vi "solar_target2.vi"(11 "Target":string) -> ()   [LabVIEW 2018]
doc: "SOLAR target demo."
uses:
  solar/solar.lvclass
  solar/solar Msg EnQ (This).vi
  solar/solar Msg UE Generate.vi
  voyager/solar_voy_def/solar_voy_def Import (Variants).vi
  solar/solar Msg Voyager (TLM).vi
  qtimer/solar_qtimer_ctl QTimer Settings.ctl
panel:
  in  "Log_Write":string="Test"
  in  "Log Write":bool
  in  "Log Pause":bool
  in  "Log Restart":bool
  in  "QTimer Start Target":bool
  in  "QTimer Stop Target":bool
  in  "QTimer Target":string
  out "QTimers":T1[](array[typedef])
  out "Subscribed DATA":variant
  out "Subscribed MSG":string
  out "Packets out":T2={"MYUINT8"={"VALUE"=255}, "MYUINT16"={"VALUE"=65535}, "MYUINT32"={"VALUE"=4294967295}, "MYUINT64"={"VALUE"=18446744073709551615}, "MYINT8"={"VALUE"=-128}, "MYINT16"={"VALUE"=-32768}, "MYINT32"={"VALUE"=-2147483648}, "MYINT64"={"VALUE"=-9223372036854775808}, "MYFLOAT32"={"VALUE"=3.141563}, "MYFLOAT64"={"VALUE"=-1.234567891e-05}, "MYSTRING"={"VALUE"="Hello World"}, "MYBLOCK"={"VALUE,t=block"="Þ­¾ï"}, "MYUINT8_ENUM"={"VALUE"=enum."ITEM2"}, "MYUINT16_ENUM"={"VALUE"=enum."BIRD"}, "MYUINT32_ENUM"={"VALUE"=enum."joe"}, "MYBOOLEAN"={"VALUE,s=OFF|ON"=FALSE}, "MYPATH"={"VALUE"=path "C:/Data/test.txt"}, "MYSTRING_FIXED"={"VALUE,b=24"="CAR"}, "MYBLOCK_FIXED"={"VALUE,t=block,b=32"="\u0001\u0002\u0003\u0004"}} {"MYFLOAT64"."VALUE" format="%#.12g"; "MYFLOAT32"."VALUE" format="%#.6g"}
  in  "Packets in":T2={"MYUINT8"={"VALUE"=255}, "MYUINT16"={"VALUE"=65535}, "MYUINT32"={"VALUE"=4294967295}, "MYUINT64"={"VALUE"=18446744073709551615}, "MYINT8"={"VALUE"=-128}, "MYINT16"={"VALUE"=-32768}, "MYINT32"={"VALUE"=-2147483648}, "MYINT64"={"VALUE"=-9223372036854775808}, "MYFLOAT32"={"VALUE"=3.141563}, "MYFLOAT64"={"VALUE"=-1.234567891e-05}, "MYSTRING"={"VALUE"="Hello World"}, "MYBLOCK"={"VALUE,t=block"="Þ­¾ï"}, "MYUINT8_ENUM"={"VALUE"=enum."ITEM2"}, "MYUINT16_ENUM"={"VALUE"=enum."BIRD"}, "MYUINT32_ENUM"={"VALUE"=enum."joe"}, "MYBOOLEAN"={"VALUE,s=OFF|ON"=FALSE}, "MYPATH"={"VALUE"=path "C:/Data/test.txt"}, "MYSTRING_FIXED"={"VALUE,b=24"="CAR"}, "MYBLOCK_FIXED"={"VALUE,t=block,b=32"="\u0001\u0002\u0003\u0004"}} {"MYFLOAT64"."VALUE" format="%#.12g"; "MYFLOAT32"."VALUE" format="%#.6g"}
  out "Time":timestamp
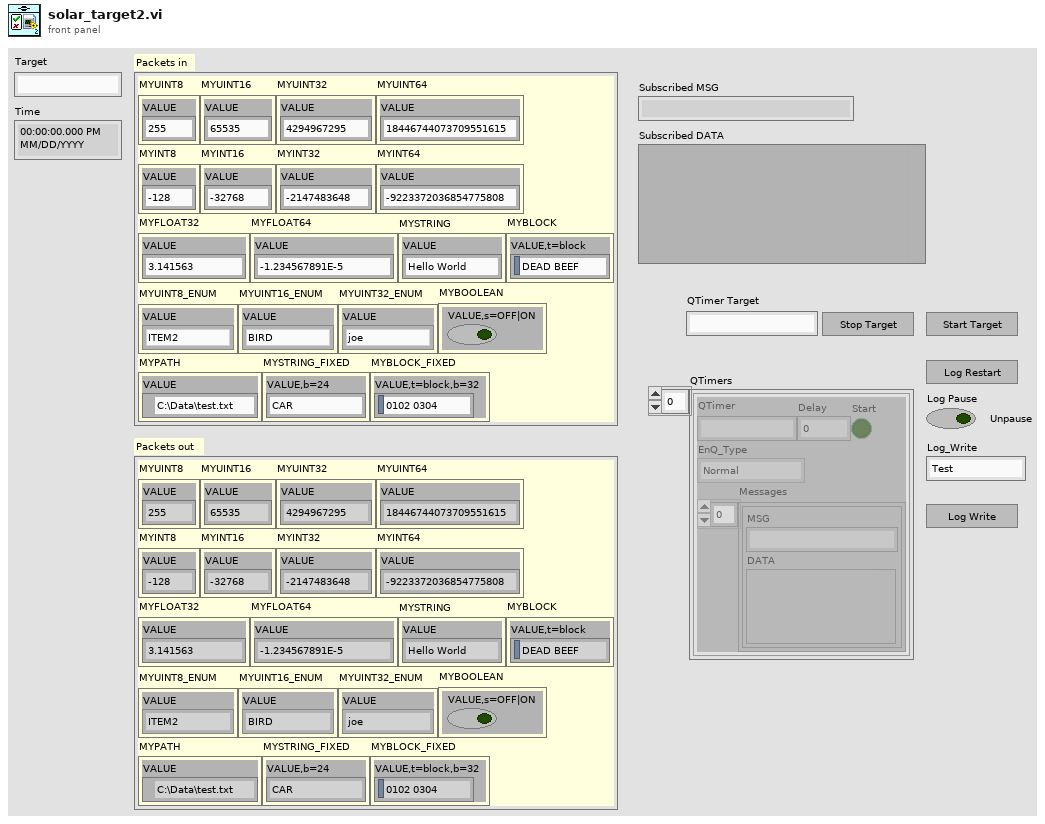
[diagram p1: front panel]
types:
  T1 = typedef "solar_qtimer_ctl QTimer Settings.ctl" = cluster{"QTimer":string, "Delay":i32, "Start":bool, "EnQ_Type":enum8{"Normal", "Priority", "IgnoreIfExists"}, "Messages":cluster{"MSG":string, "DATA":variant}[]}
  T2 = cluster{"MYUINT8":cluster{"VALUE":u8}, "MYUINT16":cluster{"VALUE":u16}, "MYUINT32":cluster{"VALUE":u32}, "MYUINT64":cluster{"VALUE":u64}, "MYINT8":cluster{"VALUE":i8}, "MYINT16":cluster{"VALUE":i16}, "MYINT32":cluster{"VALUE":i32}, "MYINT64":cluster{"VALUE":i64}, "MYFLOAT32":cluster{"VALUE":sgl}, "MYFLOAT64":cluster{"VALUE":dbl}, "MYSTRING":cluster{"VALUE":string}, "MYBLOCK":cluster{"VALUE,t=block":string}, "MYUINT8_ENUM":cluster{"VALUE":enum8{"ITEM1", "ITEM2", "ITEM3"}}, "MYUINT16_ENUM":cluster{"VALUE":enum16{"CAT", "DOG", "BIRD", "MOOSE"}}, "MYUINT32_ENUM":cluster{"VALUE":enum32{"ryan", "susan", "steve", "larry", "smith", "joe"}}, "MYBOOLEAN":cluster{"VALUE,s=OFF|ON":bool}, "MYPATH":cluster{"VALUE":path}, "MYSTRING_FIXED":cluster{"VALUE,b=24":string}, "MYBLOCK_FIXED":cluster{"VALUE,t=block,b=32":string}}
  T3 = cluster{"SIGNAL,s=NO|YES":bool, "VI,b=2048":string, "CONTROL,b=2048":string, "VALUE,t=block":string}
  T4 = cluster{"VALUE":enum8{"ITEM1", "ITEM2", "ITEM3"}}
  T5 = cluster{"VALUE":enum16{"CAT", "DOG", "BIRD", "MOOSE"}}
  T6 = cluster{"VALUE":enum32{"ryan", "susan", "steve", "larry", "smith", "joe"}}
  T7 = typedef "solar_voy_def_ctl PACKET.ctl" = cluster{"PACKET_ID":T8, "ENDIAN":enum8{"BIG", "LITTLE"}, "DESC":string, "HZRD":bool, "ITEMS":T9[], "NoExport":bool, "last_time":timestamp, "last_count":u32, "last_data":string}
  T8 = typedef "solar_voy_def_ctl PACKET_ID.ctl" = cluster{"ID":u16, "CMD":enum8{"CMD", "TLM"}, "TARGET":string, "PACKET":string}
  T9 = typedef "solar_voy_def_ctl ITEM.ctl" = cluster{"NAME":string, "OFFSET":i32, "SIZE":i32, "TYPE":T10, "EACH_SIZE":i32, "LVTYPE":T11, "MIN":dbl, "MAX":dbl, "DEFAULT":string, "DESC":string, "ID":bool, "MODIFIERS":variant, "last_value":variant}
  T10 = typedef "solar_voy_def_ctl ITEM TYPE.ctl" = enum8{"BLOCK", "INT", "UINT", "FLOAT", "STRING"}
  T11 = typedef "solar_type Item Type.ctl" = enum16{"NULL", "UNKNOWN", "CLUSTER", "I8", "I16", "I32", "I64", "U8", "U16", "U32", "U64", "U8_ENUM", "U16_ENUM", "U32_ENUM", "SGL", "DBL", "BOOLEAN", "STRING", "PATH", "VISA", "TAG", "TIME", "I8_1D", "I16_1D", "I32_1D", "I64_1D", "U8_1D", "U16_1D", "U32_1D", "U64_1D", "U8_ENUM_1D", "U16_ENUM_1D", "U32_ENUM_1D", "SGL_1D", "DBL_1D", "BOOLEAN_1D", "STRING_1D", "PATH_1D", "VISA_1D", "TAG_1D", "TIME_1D", "I8_2D", "I16_2D", "I32_2D", "I64_2D", "U8_2D", "U16_2D", "U32_2D", "U64_2D", "U8_ENUM_2D", "U16_ENUM_2D", "U32_ENUM_2D", "SGL_2D", "DBL_2D", "BOOLEAN_2D", "STRING_2D", "PATH_2D", "VISA_2D", "TAG_2D", "TIME_2D"}
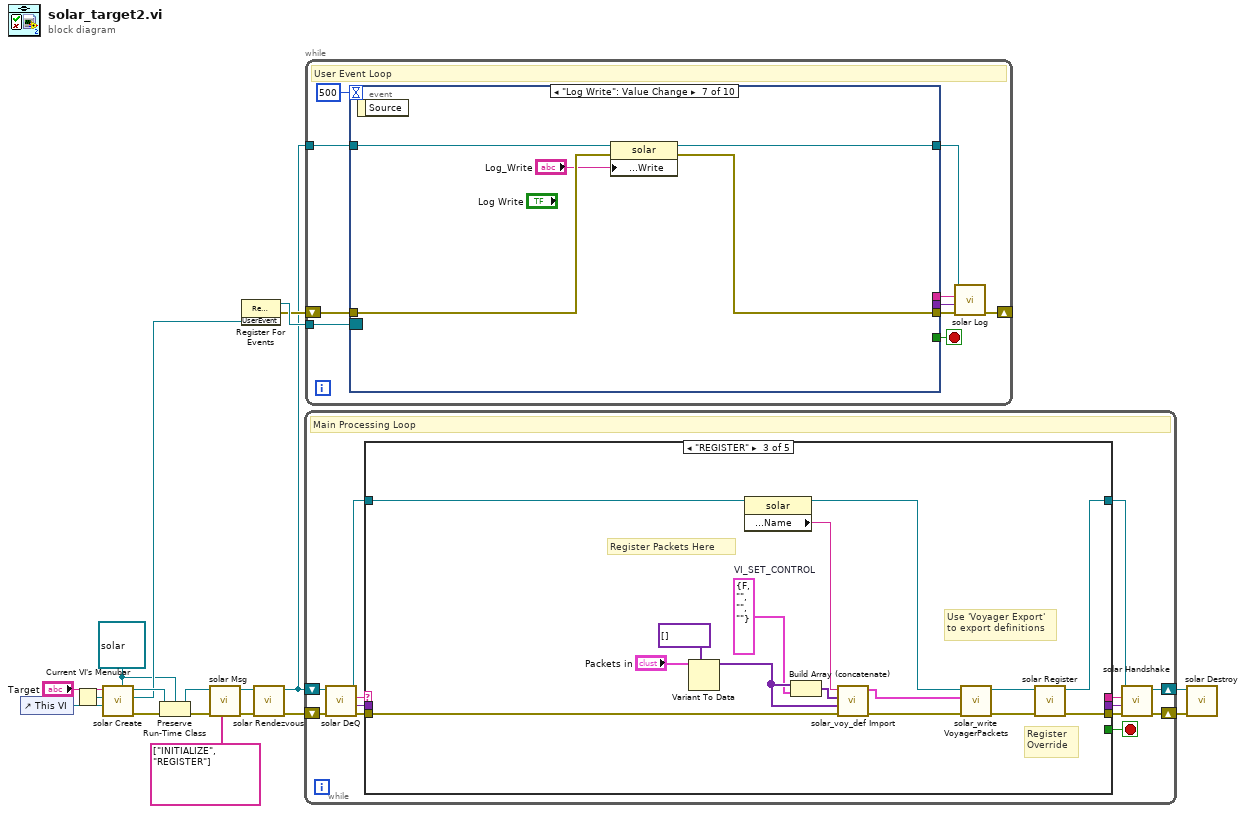
[diagram p0: block diagram]
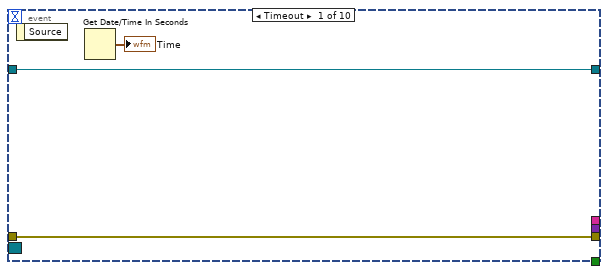
[diagram p2: hidden frame]
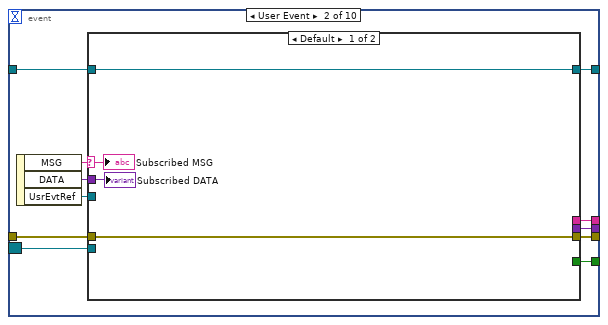
[diagram p3: hidden frame]
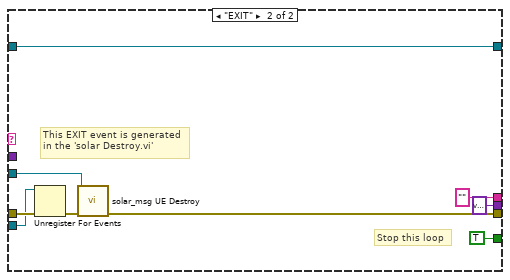
[diagram p4: hidden frame]
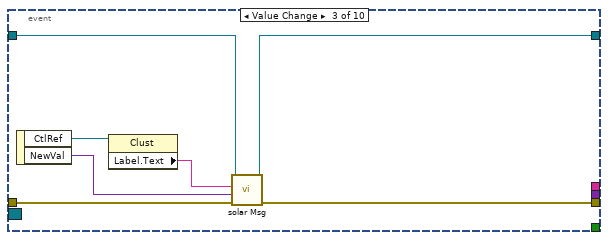
[diagram p5: hidden frame]
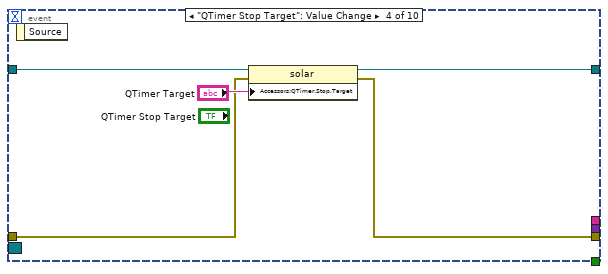
[diagram p6: hidden frame]
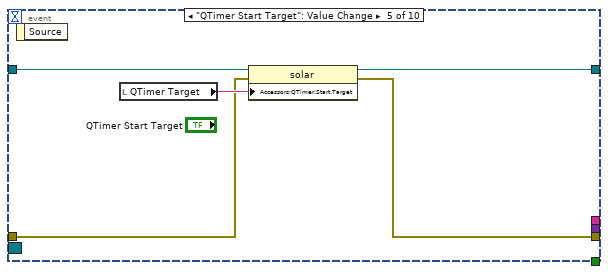
[diagram p7: hidden frame]
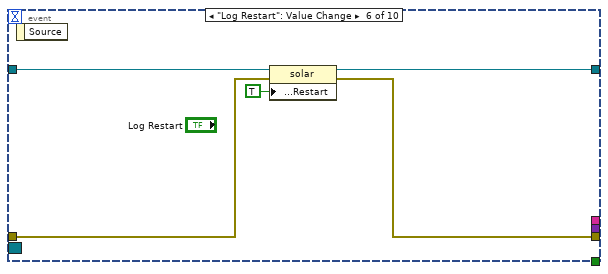
[diagram p8: hidden frame]
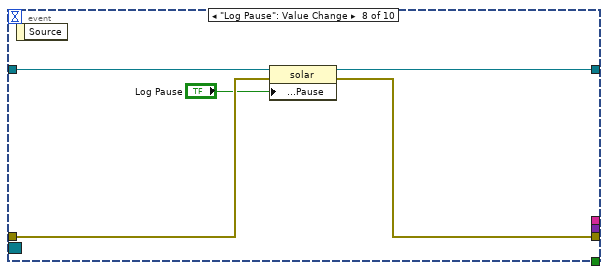
[diagram p9: hidden frame]
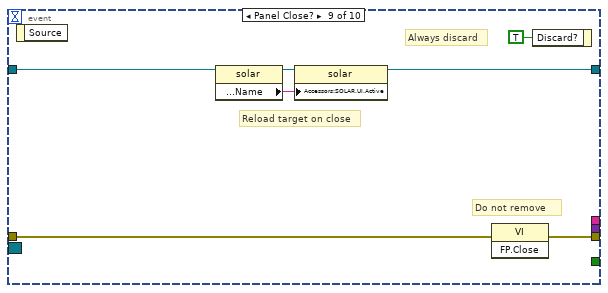
[diagram p10: hidden frame]
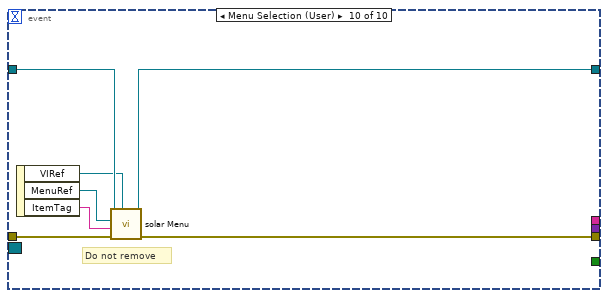
[diagram p11: hidden frame]
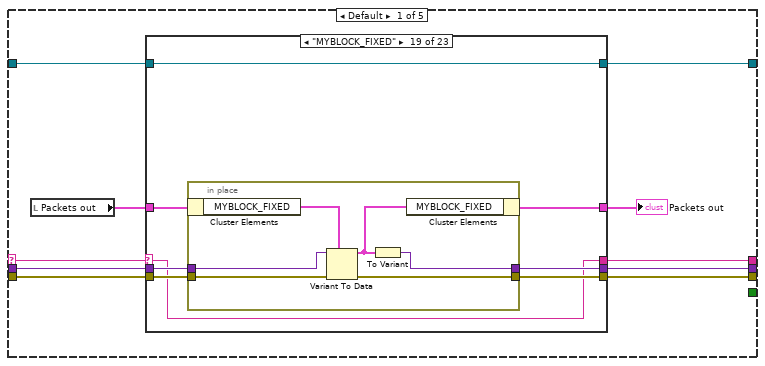
[diagram p12: hidden frame]
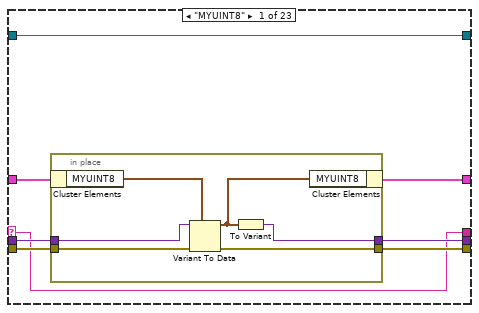
[diagram p13: hidden frame]
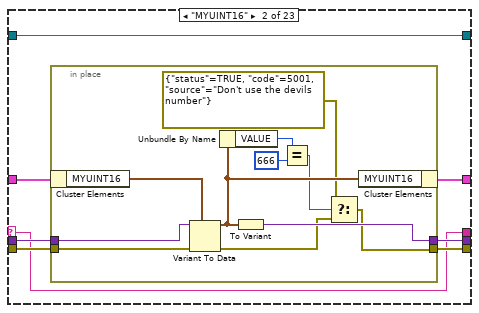
[diagram p14: hidden frame]
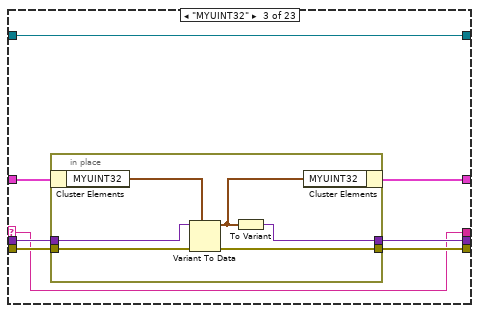
[diagram p15: hidden frame]
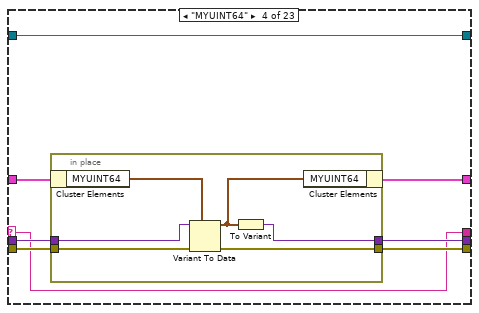
[diagram p16: hidden frame]
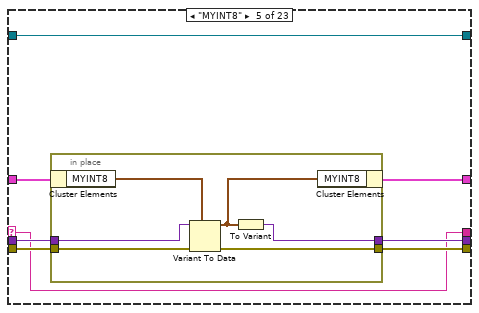
[diagram p17: hidden frame]
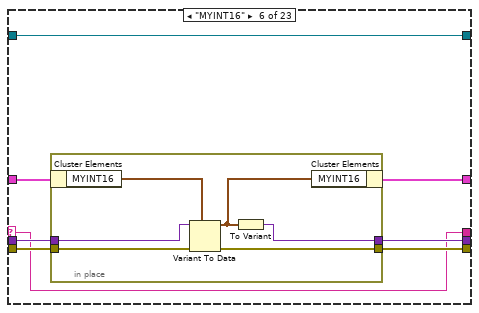
[diagram p18: hidden frame]
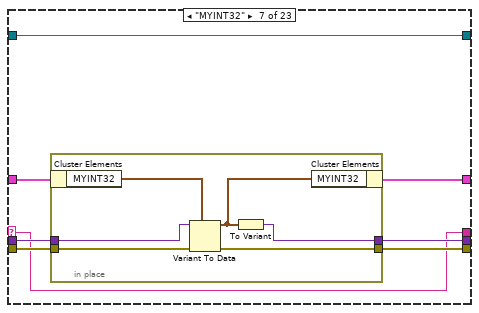
[diagram p19: hidden frame]
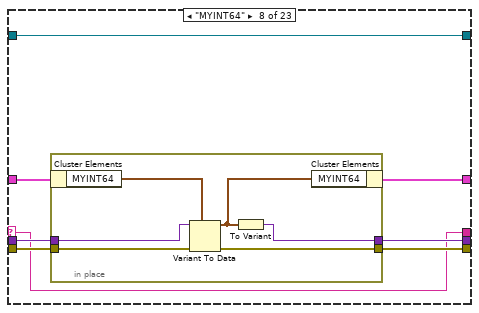
[diagram p20: hidden frame]
diagram:
  w11 = refnum<class "solar.lvclass"> refnum ("Default LVClass")
  n1 = control-ref of="This VI"() -> (w13:refnum<vi>)
  n2 = Current VI's Menubar() -> (w9:refnum<k9>)
  n3 = call "solar Create.vi"("Default LVClass"=w11, "VI Refnum"=w13, "VI MenuRef"=w9, "Target"="Target") -> ("error out"=w7:errorcluster, "UserEvent"=w14:refnum<user-event>, "solar"=w18:refnum<class "solar.lvclass">)  [unwired: 4 in, 1 out]
  n4 = Preserve Run-Time Class(object in=w18, error in=w7, 2:w11) -> (object out=w2:refnum<class "solar.lvclass">, error out=w3:errorcluster)
  n5 = call-poly "solar Msg.vi"("MSG Array"=string[] ["INITIALIZE", "REGISTER"] ("Script (\"PACKET{ITEM:VAL}\")"), "error in (no error)"=w3, "solar in"=w2) -> ("error out"=w6:errorcluster, "solar out"=w4:refnum<class "solar.lvclass">)  [unwired: 6 in, 1 out]
  n6 = register-events(w14) -> (reference out=w15:refnum<event-registration>, error out=w8:errorcluster)  [unwired: 2 in]
  n7 = call-dynamic "solar Rendezvous.vi"("error in (no error)"=w6, "solar in"=w4) -> ("error out"=w5:errorcluster, "solar out"=w1:refnum<class "solar.lvclass">)  [unwired: 6 in, 2 out]
  n8 = while {
    shift-right: [w28] -> w17
    shift-left: w5 -> [w30]
    shift-right: [w24] -> w16
    shift-left: w1 -> [w31]
    stop <- w23 stop-if-true
    # "Main Processing Loop"
    n9 = call "solar DeQ.vi"("error in (no error)"=w30, "solar in"=w31) -> ("error out"=w29:errorcluster, "DATA"=w19:variant, "MSG"=w20:string, "solar out"=w25:refnum<class "solar.lvclass">)  [unwired: 5 in, 1 out]
    n10 = case shown="\"REGISTER\"" w20 {
      selector: w20 -> [w36 _ _ _ _]
      tunnel: [w41 w367 w380 w386 w404] -> w27
      tunnel: w29 -> [w34 w360 w382 w390 w404]
      tunnel: [w39 w366 w379 w385 w405] -> w26
      tunnel: w25 -> [w40 w363 w373 w389 w405]
      tunnel: w19 -> [w35 _ _ _ _]
      tunnel: [_ _ _ w383 _] -> w23
      tunnel: [w38 _ _ _ _] -> w22
      tunnel: [w37 _ _ _ _] -> w21
      frame Default {
        n11 = local read "Packets out"() -> (w32:T2)
        n12 = case shown="\"MYBLOCK_FIXED\"" w36 {
          selector: w36 -> [w44 w58 w77 w91 w105 w119 w133 w147 w161 w175 w189 w203 w217 w231 w245 w259 w273 w287 w301 _ _ _ w338]
          tunnel: [w46 w60 w79 w93 w107 w121 w135 w149 w163 w177 w191 w205 w219 w233 w247 w261 w275 w289 w303 w315 w323 w330 w343] -> w41
          tunnel: w40 -> [w49 w63 w82 w96 w110 w124 w138 w152 w166 w180 w194 w208 w222 w236 w250 w264 w278 w292 w306 w319 w322 w329 w342]
          tunnel: [w49 w63 w82 w96 w110 w124 w138 w152 w166 w180 w194 w208 w222 w236 w250 w264 w278 w292 w306 w319 w321 w328 w341] -> w39
          tunnel: [w44 w58 w77 w91 w105 w119 w133 w147 w161 w175 w189 w203 w217 w231 w245 w259 w273 w287 w301 _ _ _ w340] -> w38
          tunnel: [w45 w59 w78 w92 w106 w120 w134 w148 w162 w176 w190 w204 w218 w232 w246 w260 w274 w288 w302 _ _ _ w339] -> w37
          tunnel: w35 -> [w47 w61 w80 w94 w108 w122 w136 w150 w164 w178 w192 w206 w220 w234 w248 w262 w276 w290 w304 w316 _ _ w337]
          tunnel: w34 -> [w48 w62 w81 w95 w109 w123 w137 w151 w165 w179 w193 w207 w221 w235 w249 w263 w277 w291 w305 w318 w324 w331 w336]
          tunnel: [w42 w56 w75 w89 w103 w117 w131 w145 w159 w173 w187 w201 w215 w229 w243 w257 w271 w285 w299 w320 w327 w334 w335] -> w33
          tunnel: w32 -> [w43 w57 w76 w90 w104 w118 w132 w146 w160 w174 w188 w202 w216 w230 w244 w258 w272 w286 w300 w320 w327 w334 w335]
          frame "MYUINT8" {
            n13 = in-place {
              in-place-border: w48 -> [w55]
              in-place-border: w47 -> [w54]
              in-place-border: [w51] -> w46
              in-place-border: [w50] -> w45
              n14 = in-place-cluster #1(w43) -> ("MYUINT8"=w53:cluster{"VALUE":u8})
              n15 = Variant To Data(error in=w55, type=w53, Variant=w54) -> (data=w52:cluster{"VALUE":u8}, error out=w51:errorcluster)
              n16 = To Variant(anything=w52) -> (Variant=w50:variant)
              n17 = in-place-cluster #1("MYUINT8"=w52) -> (w42:T2)
            }
          }
          frame "MYUINT16" {
            n18 = in-place {
              in-place-border: w62 -> [w74]
              in-place-border: w61 -> [w73]
              in-place-border: [w65] -> w60
              in-place-border: [w71] -> w59
              n19 = in-place-cluster #2(w57) -> ("MYUINT16"=w72:cluster{"VALUE":u16})
              n20 = Variant To Data(error in=w74, type=w72, Variant=w73) -> (data=w70:cluster{"VALUE":u16}, error out=w66:errorcluster)
              n21 = Unbundle By Name(w70) -> ("VALUE"=w69:u16)
              n22 = To Variant(anything=w70) -> (Variant=w71:variant)
              n23 = Equal?(x=w69, y=u16 666 ("VALUE")) -> (x = y?=w67:bool)
              n24 = Select(t=errorcluster {"status"=TRUE, "code"=5001, "source"="Don't use the devils number"}, s=w67, f=w66) -> (s? t:f=w65:errorcluster)
              n25 = in-place-cluster #2("MYUINT16"=w70) -> (w56:T2)
            }
          }
          frame "MYUINT32" {
            n26 = in-place {
              in-place-border: w81 -> [w88]
              in-place-border: w80 -> [w87]
              in-place-border: [w84] -> w79
              in-place-border: [w83] -> w78
              n27 = in-place-cluster #3(w76) -> ("MYUINT32"=w86:cluster{"VALUE":u32})
              n28 = Variant To Data(error in=w88, type=w86, Variant=w87) -> (data=w85:cluster{"VALUE":u32}, error out=w84:errorcluster)
              n29 = To Variant(anything=w85) -> (Variant=w83:variant)
              n30 = in-place-cluster #3("MYUINT32"=w85) -> (w75:T2)
            }
          }
          frame "MYUINT64" {
            n31 = in-place {
              in-place-border: w95 -> [w102]
              in-place-border: w94 -> [w101]
              in-place-border: [w98] -> w93
              in-place-border: [w97] -> w92
              n32 = in-place-cluster #4(w90) -> ("MYUINT64"=w100:cluster{"VALUE":u64})
              n33 = Variant To Data(error in=w102, type=w100, Variant=w101) -> (data=w99:cluster{"VALUE":u64}, error out=w98:errorcluster)
              n34 = To Variant(anything=w99) -> (Variant=w97:variant)
              n35 = in-place-cluster #4("MYUINT64"=w99) -> (w89:T2)
            }
          }
          frame "MYINT8" {
            n36 = in-place {
              in-place-border: w109 -> [w116]
              in-place-border: w108 -> [w115]
              in-place-border: [w112] -> w107
              in-place-border: [w111] -> w106
              n37 = in-place-cluster #5(w104) -> ("MYINT8"=w114:cluster{"VALUE":i8})
              n38 = Variant To Data(error in=w116, type=w114, Variant=w115) -> (data=w113:cluster{"VALUE":i8}, error out=w112:errorcluster)
              n39 = To Variant(anything=w113) -> (Variant=w111:variant)
              n40 = in-place-cluster #5("MYINT8"=w113) -> (w103:T2)
            }
          }
          frame "MYINT16" {
            n41 = in-place {
              in-place-border: w123 -> [w130]
              in-place-border: w122 -> [w129]
              in-place-border: [w126] -> w121
              in-place-border: [w125] -> w120
              n42 = in-place-cluster #6(w118) -> ("MYINT16"=w128:cluster{"VALUE":i16})
              n43 = Variant To Data(error in=w130, type=w128, Variant=w129) -> (data=w127:cluster{"VALUE":i16}, error out=w126:errorcluster)
              n44 = To Variant(anything=w127) -> (Variant=w125:variant)
              n45 = in-place-cluster #6("MYINT16"=w127) -> (w117:T2)
            }
          }
          frame "MYINT32" {
            n46 = in-place {
              in-place-border: w137 -> [w144]
              in-place-border: w136 -> [w143]
              in-place-border: [w140] -> w135
              in-place-border: [w139] -> w134
              n47 = in-place-cluster #7(w132) -> ("MYINT32"=w142:cluster{"VALUE":i32})
              n48 = Variant To Data(error in=w144, type=w142, Variant=w143) -> (data=w141:cluster{"VALUE":i32}, error out=w140:errorcluster)
              n49 = To Variant(anything=w141) -> (Variant=w139:variant)
              n50 = in-place-cluster #7("MYINT32"=w141) -> (w131:T2)
            }
          }
          frame "MYINT64" {
            n51 = in-place {
              in-place-border: w151 -> [w158]
              in-place-border: w150 -> [w157]
              in-place-border: [w154] -> w149
              in-place-border: [w153] -> w148
              n52 = in-place-cluster #8(w146) -> ("MYINT64"=w156:cluster{"VALUE":i64})
              n53 = Variant To Data(error in=w158, type=w156, Variant=w157) -> (data=w155:cluster{"VALUE":i64}, error out=w154:errorcluster)
              n54 = To Variant(anything=w155) -> (Variant=w153:variant)
              n55 = in-place-cluster #8("MYINT64"=w155) -> (w145:T2)
            }
          }
          frame "MYFLOAT32" {
            n56 = in-place {
              in-place-border: w165 -> [w172]
              in-place-border: w164 -> [w171]
              in-place-border: [w168] -> w163
              in-place-border: [w167] -> w162
              n57 = in-place-cluster #9(w160) -> ("MYFLOAT32"=w170:cluster{"VALUE":sgl})
              n58 = Variant To Data(error in=w172, type=w170, Variant=w171) -> (data=w169:cluster{"VALUE":sgl}, error out=w168:errorcluster)
              n59 = To Variant(anything=w169) -> (Variant=w167:variant)
              n60 = in-place-cluster #9("MYFLOAT32"=w169) -> (w159:T2)
            }
          }
          frame "MYFLOAT64" {
            n61 = in-place {
              in-place-border: w179 -> [w186]
              in-place-border: w178 -> [w185]
              in-place-border: [w182] -> w177
              in-place-border: [w181] -> w176
              n62 = in-place-cluster #10(w174) -> ("MYFLOAT64"=w184:cluster{"VALUE":dbl})
              n63 = Variant To Data(error in=w186, type=w184, Variant=w185) -> (data=w183:cluster{"VALUE":dbl}, error out=w182:errorcluster)
              n64 = To Variant(anything=w183) -> (Variant=w181:variant)
              n65 = in-place-cluster #10("MYFLOAT64"=w183) -> (w173:T2)
            }
          }
          frame "MYSTRING" {
            n66 = in-place {
              in-place-border: w193 -> [w200]
              in-place-border: w192 -> [w199]
              in-place-border: [w196] -> w191
              in-place-border: [w195] -> w190
              n67 = in-place-cluster #11(w188) -> ("MYSTRING"=w198:cluster{"VALUE":string})
              n68 = Variant To Data(error in=w200, type=w198, Variant=w199) -> (data=w197:cluster{"VALUE":string}, error out=w196:errorcluster)
              n69 = To Variant(anything=w197) -> (Variant=w195:variant)
              n70 = in-place-cluster #11("MYSTRING"=w197) -> (w187:T2)
            }
          }
          frame "MYBLOCK" {
            n71 = in-place {
              in-place-border: w207 -> [w214]
              in-place-border: w206 -> [w213]
              in-place-border: [w210] -> w205
              in-place-border: [w209] -> w204
              n72 = in-place-cluster #12(w202) -> ("MYBLOCK"=w212:cluster{"VALUE,t=block":string})
              n73 = Variant To Data(error in=w214, type=w212, Variant=w213) -> (data=w211:cluster{"VALUE,t=block":string}, error out=w210:errorcluster)
              n74 = To Variant(anything=w211) -> (Variant=w209:variant)
              n75 = in-place-cluster #12("MYBLOCK"=w211) -> (w201:T2)
            }
          }
          frame "MYUINT8_ENUM" {
            n76 = in-place {
              in-place-border: w221 -> [w228]
              in-place-border: w220 -> [w227]
              in-place-border: [w224] -> w219
              in-place-border: [w223] -> w218
              n77 = in-place-cluster #13(w216) -> ("MYUINT8_ENUM"=w226:T4)
              n78 = Variant To Data(error in=w228, type=w226, Variant=w227) -> (data=w225:T4, error out=w224:errorcluster)
              n79 = To Variant(anything=w225) -> (Variant=w223:variant)
              n80 = in-place-cluster #13("MYUINT8_ENUM"=w225) -> (w215:T2)
            }
          }
          frame "MYUINT16_ENUM" {
            n81 = in-place {
              in-place-border: w235 -> [w242]
              in-place-border: w234 -> [w241]
              in-place-border: [w238] -> w233
              in-place-border: [w237] -> w232
              n82 = in-place-cluster #14(w230) -> ("MYUINT16_ENUM"=w240:T5)
              n83 = Variant To Data(error in=w242, type=w240, Variant=w241) -> (data=w239:T5, error out=w238:errorcluster)
              n84 = To Variant(anything=w239) -> (Variant=w237:variant)
              n85 = in-place-cluster #14("MYUINT16_ENUM"=w239) -> (w229:T2)
            }
          }
          frame "MYUINT32_ENUM" {
            n86 = in-place {
              in-place-border: w249 -> [w256]
              in-place-border: w248 -> [w255]
              in-place-border: [w252] -> w247
              in-place-border: [w251] -> w246
              n87 = in-place-cluster #15(w244) -> ("MYUINT32_ENUM"=w254:T6)
              n88 = Variant To Data(error in=w256, type=w254, Variant=w255) -> (data=w253:T6, error out=w252:errorcluster)
              n89 = To Variant(anything=w253) -> (Variant=w251:variant)
              n90 = in-place-cluster #15("MYUINT32_ENUM"=w253) -> (w243:T2)
            }
          }
          frame "MYBOOLEAN" {
            n91 = in-place {
              in-place-border: w263 -> [w270]
              in-place-border: w262 -> [w269]
              in-place-border: [w266] -> w261
              in-place-border: [w265] -> w260
              n92 = in-place-cluster #16(w258) -> ("MYBOOLEAN"=w268:cluster{"VALUE,s=OFF|ON":bool})
              n93 = Variant To Data(error in=w270, type=w268, Variant=w269) -> (data=w267:cluster{"VALUE,s=OFF|ON":bool}, error out=w266:errorcluster)
              n94 = To Variant(anything=w267) -> (Variant=w265:variant)
              n95 = in-place-cluster #16("MYBOOLEAN"=w267) -> (w257:T2)
            }
          }
          frame "MYPATH" {
            n96 = in-place {
              in-place-border: w277 -> [w284]
              in-place-border: w276 -> [w283]
              in-place-border: [w280] -> w275
              in-place-border: [w279] -> w274
              n97 = in-place-cluster #17(w272) -> ("MYPATH"=w282:cluster{"VALUE":path})
              n98 = Variant To Data(error in=w284, type=w282, Variant=w283) -> (data=w281:cluster{"VALUE":path}, error out=w280:errorcluster)
              n99 = To Variant(anything=w281) -> (Variant=w279:variant)
              n100 = in-place-cluster #17("MYPATH"=w281) -> (w271:T2)
            }
          }
          frame "MYSTRING_FIXED" {
            n101 = in-place {
              in-place-border: w291 -> [w298]
              in-place-border: w290 -> [w297]
              in-place-border: [w294] -> w289
              in-place-border: [w293] -> w288
              n102 = in-place-cluster #18(w286) -> ("MYSTRING_FIXED"=w296:cluster{"VALUE,b=24":string})
              n103 = Variant To Data(error in=w298, type=w296, Variant=w297) -> (data=w295:cluster{"VALUE,b=24":string}, error out=w294:errorcluster)
              n104 = To Variant(anything=w295) -> (Variant=w293:variant)
              n105 = in-place-cluster #18("MYSTRING_FIXED"=w295) -> (w285:T2)
            }
          }
          frame "MYBLOCK_FIXED" {
            n106 = in-place {
              in-place-border: w305 -> [w312]
              in-place-border: w304 -> [w311]
              in-place-border: [w308] -> w303
              in-place-border: [w307] -> w302
              n107 = in-place-cluster #19(w300) -> ("MYBLOCK_FIXED"=w310:cluster{"VALUE,t=block,b=32":string})
              n108 = Variant To Data(error in=w312, type=w310, Variant=w311) -> (data=w309:cluster{"VALUE,t=block,b=32":string}, error out=w308:errorcluster)
              n109 = To Variant(anything=w309) -> (Variant=w307:variant)
              n110 = in-place-cluster #19("MYBLOCK_FIXED"=w309) -> (w299:T2)
            }
          }
          frame "VI_SET_CONTROL" {
            n111 = Variant To Data(error in=w318, type=T3 {"SIGNAL,s=NO|YES"=FALSE, "VI,b=2048"="", "CONTROL,b=2048"="", "VALUE,t=block"=""} ("VI_SET_CONTROL"), Variant=w316) -> (data=w313:T3, error out=w317:errorcluster)
            n112 = call "solar_voy Set VI Control.vi"("error in (no error)"=w317, "VI_SET_CONTROL"=w313) -> ("error out"=w315:errorcluster)  [unwired: 9 in]
          }
          frame "SendError" {
            n113 = call-poly "solar Msg.vi"("error in (no error)"=w324, "TLM_DATA (No HDR)"=errorcluster {"status"=TRUE, "code"=9234, "source"="Bad aasfd error test"} ("t"), "TLM"="ERROR", "solar in"=w322) -> ("error out"=w323:errorcluster, "solar out"=w321:refnum<class "solar.lvclass">)  [unwired: 6 in]
          }
          frame "SendWarning" {
            n114 = call-poly "solar Msg.vi"("error in (no error)"=w331, "TLM_DATA (No HDR)"=errorcluster {"status"=FALSE, "code"=9235, "source"="Bad aasfd warning test"} ("t"), "TLM"="ERROR", "solar in"=w329) -> ("error out"=w330:errorcluster, "solar out"=w328:refnum<class "solar.lvclass">)  [unwired: 6 in]
          }
          frame Default {
            # "Command\nOverride"
            n115 = call-dynamic "solar Command.vi"("error in (no error)"=w336, "CMD_DATA"=w337, "CMD"=w338, "solar in"=w342) -> ("error out"=w343:errorcluster, "TLM_DATA"=w339:variant, "TLM"=w340:string, "solar out"=w341:refnum<class "solar.lvclass">)  [unwired: 3 in, 1 out]
          }
        }
        "Packets out" <- w33
      }
      frame "INITIALIZE" {
        # "Subscribe all telemetry to return\nin This User Event"
        # "Wire temporary\nControl refnums\nhere"
        # "Load Temp\nControls"
        # "Initialize\nOverride"
        # "Initialize\nTarget\nHere"
        n116 = property class="solar"(reference=w363, error in=w360) -> (reference out=w361:refnum<class "solar.lvclass">, error out=w358:errorcluster, "Accessors:This.Name"=w344:string)
        n117 = Random Number (0-1)() -> (number: 0 to 1=w349:dbl)
        n118 = Concatenate Strings(w344, "_READ" ("string")) -> (w346:string)
        n119 = Bundle("number: 0 to 1"=w349) -> (w348:cluster{"number: 0 to 1":dbl})  [unwired: 1 in]
        n120 = Bundle By Name(cluster=cluster{"MSG":string, "DATA":variant} {"MSG"="", "DATA"=variant} ("Message"), "MSG"=w346, "DATA"=w348) -> (w351:cluster{"MSG":string, "DATA":variant})
        n121 = Build Array(w351) -> (w350:cluster{"MSG":string, "DATA":variant}[])
        n122 = Bundle By Name(cluster=T1 {"QTimer"="", "Delay"=0, "Start"=FALSE, "EnQ_Type"=enum."IgnoreIfExists", "Messages"=[]} ("QTimer:Add"), "QTimer"=w344, "Delay"=1000, "Start"=TRUE, "EnQ_Type"=enum8{"Normal", "Priority", "IgnoreIfExists"}."IgnoreIfExists", "Messages"=w350) -> (w356:T1)
        n123 = property class="solar"(reference=w361, error in=w358, "Accessors:Subscribe.ThisUE2Dest"=w344, "Accessors:QTimer.Add"=w356) -> (reference out=w362:refnum<class "solar.lvclass">, error out=w359:errorcluster, "Accessors:QTimer.QTimers"=→"QTimers":T1[])
        n124 = call "solar Ctrls Load.vi"("error in (no error)"=w359, "solar in"=w362) -> ("error out"=w365:errorcluster, "solar out"=w364:refnum<class "solar.lvclass">)  [unwired: 8 in]
        n125 = call-dynamic "solar Initialize.vi"("error in (no error)"=w365, "solar in"=w364) -> ("error out"=w367:errorcluster, "solar out"=w366:refnum<class "solar.lvclass">)  [unwired: 8 in]
      }
      frame "REGISTER" {
        w374 = T3 {"SIGNAL,s=NO|YES"=FALSE, "VI,b=2048"="", "CONTROL,b=2048"="", "VALUE,t=block"=""}  # VI_SET_CONTROL
        # "Use 'Voyager Export'\nto export definitions"
        # "Register\nOverride"
        # "Register Packets Here"
        n126 = Variant To Data(type=variant[] [], Variant="Packets in") -> (data=w376:variant[])  [unwired: 1 in, 1 out]
        n127 = property class="solar"(reference=w373) -> (reference out=w370:refnum<class "solar.lvclass">, "Accessors:This.Name"=w381:string)  [unwired: 1 in, 1 out]
        n128 = Build Array (concatenate)(w376, w374) -> (w375:variant[])
        n129 = call-poly "solar_voy_def Import.vi"("error in (no error)"=w382, "TLMs"=w376, "CMDs"=w375, "TARGET"=w381) -> ("error out"=w371:errorcluster, "PACKETS"=w369:T7[])  [unwired: 6 in]
        n130 = call "solar_write VoyagerPackets.vi"("error in (no error)"=w371, "PACKETS"=w369, "solar in"=w370) -> ("error out"=w372:errorcluster, "solar out"=w368:refnum<class "solar.lvclass">)  [unwired: 7 in]
        n131 = call-dynamic "solar Register.vi"("error in (no error)"=w372, "solar in"=w368) -> ("error out"=w380:errorcluster, "solar out"=w379:refnum<class "solar.lvclass">)  [unwired: 8 in]
      }
      frame "EXIT" {
        # "Exit\nOverride"
        n132 = call-dynamic "solar Exit.vi"("error in (no error)"=w390, "solar in"=w389) -> ("error out"=w387:errorcluster, "Exit?"=w384:bool, "solar out"=w388:refnum<class "solar.lvclass">)  [unwired: 7 in]
        n133 = case shown="True" w384 {
          tunnel: w388 -> [w393 w398]
          tunnel: w387 -> [w392 w397]
          tunnel: [w392 w396] -> w386
          tunnel: [w393 w395] -> w385
          tunnel: [FALSE ("EXIT") w394] -> w383
          frame False {
            # "Do not exit target"
            # "EXIT ABORTED\n- Execute shutdown sequence override"
          }
          frame True {
            w394 = TRUE  # EXIT
            # "Save Temp\nControls"
            # "Send 'EXIT' to\n User Event"
            # "Send 'EXIT' to\n all children"
            n134 = call "solar Exit (Children).vi"("error in (no error)"=w397, "solar in"=w398) -> ("error out"=w400:errorcluster, "solar out"=w399:refnum<class "solar.lvclass">)  [unwired: 8 in]
            n135 = call-poly "solar Msg.vi"("error in (no error)"=w400, "MSG (last)"="EXIT" ("MSG (Last)"), "solar in"=w399) -> ("error out"=w402:errorcluster, "solar out"=w401:refnum<class "solar.lvclass">)  [unwired: 7 in]
            n136 = call "solar Ctrls Save.vi"("error in (no error)"=w402, "solar in"=w401) -> ("error out"=w396:errorcluster, "solar out"=w395:refnum<class "solar.lvclass">)  [unwired: 7 in, 1 out]
          }
        }
      }
      frame "EMERGENCY_STOP" {
        # "If Main Target: Handle emergency conditions here\nIf Child Target: Ignore"
      }
    }
    n137 = call "solar Handshake.vi"("error in (no error)"=w27, "TLM_DATA"=w21, "TLM"=w22, "solar in"=w26) -> ("error out"=w28:errorcluster, "solar out"=w24:refnum<class "solar.lvclass">)  [unwired: 6 in]
  }
  n138 = while {
    shift-right: [w409] -> _
    shift-left: w8 -> [w414]
    tunnel: w15 -> [w415]
    tunnel: w1 -> [w412]
    stop <- w413 stop-if-true
    # "User Event Loop"
    n139 = event shown="[6] \"Log Write\": Value Change" {
      selector: w415 -> [_ w426 _ _ _ _ _ _ _ _]
      dyn-events: _ -> [_ _ _ _ _ _ _ _ _ _]
      timeout: 500 -> [_ _ _ _ _ _ _ _ _ _]
      tunnel: w414 -> [w418 w427 w449 w451 w455 w461 w466 w471 w480 w488]
      tunnel: [w418 w428 w448 w450 w456 w462 w467 w472 w479 w487] -> w411
      tunnel: [_ w425 _ _ _ _ _ _ _ _] -> w413
      tunnel: w412 -> [w416 w420 w447 w454 w459 w464 w469 w474 w478 w484]
      tunnel: [_ w423 _ _ _ _ _ _ _ _] -> w408
      tunnel: [w416 w421 w446 w453 w458 w463 w468 w473 w476 w483] -> w410
      tunnel: [_ w419 _ _ _ _ _ _ _ _] -> w407
      event Timeout {
        n140 = event-data() -> ()  [unwired: 1 in, 1 out]
        n141 = Get Date/Time In Seconds() -> (seconds since 1Jan1904=→"Time":timestamp)
      }
      event User Event {
        n142 = event-data() -> ("MSG"=w429:string, "DATA"=w424:variant, "UsrEvtRef"=w422:refnum<user-event>)  [unwired: 1 in]
        n143 = case shown="Default" w429 {
          selector: w429 -> [w431 _]
          tunnel: [w433 w441] -> w428
          tunnel: w427 -> [w433 w442]
          tunnel: w426 -> [_ w438]
          tunnel: w422 -> [_ w440]
          tunnel: [_ TRUE] -> w425
          tunnel: w424 -> [w430 _]
          tunnel: [_ ""] -> w423
          tunnel: [w432 w435] -> w421
          tunnel: w420 -> [w432 w435]
          tunnel: [_ variant] -> w419
          frame Default {
            "Subscribed MSG" <- w431
            "Subscribed DATA" <- w430
          }
          frame "EXIT" {
            # "Stop this loop"
            # "This EXIT event is generated\nin the 'solar Destroy.vi'"
            n144 = Unregister For Events(event registration refnum=w438, error in=w442) -> (error out=w439:errorcluster)
            n145 = call "solar_msg UE Destroy.vi"("error in (no error)"=w439, "UserEvent"=w440) -> ("error out"=w441:errorcluster)  [unwired: 9 in]
          }
        }
      }
      event "Packets in.MYUINT8", "Packets in.MYUINT16", "Packets in.MYUINT32", "Packets in.MYUINT64", "Packets in.MYINT8", "Packets in.MYINT16", "Packets in.MYINT32", "Packets in.MYINT64", "Packets in.MYFLOAT32", "Packets in.MYFLOAT64", "Packets in.MYSTRING", "Packets in.MYBLOCK", "Packets in.MYUINT8_ENUM", "Packets in.MYUINT16_ENUM", "Packets in.MYUINT32_ENUM", "Packets in.MYBOOLEAN", "Packets in.MYPATH", "Packets in.MYSTRING_FIXED", "Packets in.MYBLOCK_FIXED": Value Change {
        n146 = event-data() -> ("CtlRef"=w444:refnum<vi>, "NewVal"=w445:variant)  [unwired: 1 in]
        n147 = property class="Clust"(reference=w444) -> ("Label.Text"=w443:string)  [unwired: 1 in, 2 out]
        n148 = call-poly "solar Msg.vi"("error in (no error)"=w449, "DATA (last)"=w445, "MSG (last)"=w443, "solar in"=w447) -> ("error out"=w448:errorcluster, "solar out"=w446:refnum<class "solar.lvclass">)  [unwired: 5 in, 1 out]
      }
      event "QTimer Stop Target": Value Change {
        n149 = event-data() -> ()  [unwired: 1 in, 1 out]
        n150 = property class="solar"(reference=w454, error in=w451, "Accessors:QTimer.Stop.Target"="QTimer Target") -> (reference out=w453:refnum<class "solar.lvclass">, error out=w450:errorcluster)
      }
      event "QTimer Start Target": Value Change {
        n151 = event-data() -> ()  [unwired: 1 in, 1 out]
        n152 = local read "QTimer Target"() -> (w457:string)
        n153 = property class="solar"(reference=w459, error in=w455, "Accessors:QTimer.Start.Target"=w457) -> (reference out=w458:refnum<class "solar.lvclass">, error out=w456:errorcluster)
      }
      event "Log Restart": Value Change {
        n154 = event-data() -> ()  [unwired: 1 in, 1 out]
        n155 = property class="solar"(reference=w464, error in=w461, "Accessors:Log.Restart"=TRUE ("Log:Restart")) -> (reference out=w463:refnum<class "solar.lvclass">, error out=w462:errorcluster)
      }
      event "Log Write": Value Change {
        n156 = event-data() -> ()  [unwired: 1 in, 1 out]
        n157 = property class="solar"(reference=w469, error in=w466, "Accessors:Log.Write"="Log_Write") -> (reference out=w468:refnum<class "solar.lvclass">, error out=w467:errorcluster)
      }
      event "Log Pause": Value Change {
        n158 = event-data() -> ()  [unwired: 1 in, 1 out]
        n159 = property class="solar"(reference=w474, error in=w471, "Accessors:Log.Pause"="Log Pause") -> (reference out=w473:refnum<class "solar.lvclass">, error out=w472:errorcluster)
      }
      event Panel Close? {
        # "Do not remove"
        # "Reload target on close"
        # "Always discard"
        n160 = event-data() -> ()  [unwired: 1 in, 1 out]
        n161 = property class="solar"(reference=w478) -> (reference out=w477:refnum<class "solar.lvclass">, "Accessors:This.Name"=w475:string)  [unwired: 1 in, 1 out]
        n162 = property class="solar"(reference=w477, "Accessors:SOLAR.UI.Active"=w475) -> (reference out=w476:refnum<class "solar.lvclass">)  [unwired: 1 in, 1 out]
        n163 = invoke class="VI" method="FP.Close"(error in=w480) -> (error out=w479:errorcluster)  [unwired: 2 in, 2 out]
        n164 = event-data("Discard?"=TRUE) -> ()  [unwired: 1 in, 1 out]
      }
      event Menu Selection (User) {
        # "Do not remove"
        n165 = event-data() -> ("VIRef"=w482:refnum<vi>, "MenuRef"=w485:refnum<k9>, "ItemTag"=w486:string)  [unwired: 1 in]
        n166 = call "solar Menu.vi"("VIRef"=w482, "error in (no error)"=w488, "ItemTag"=w486, "MenuRef"=w485, "solar in"=w484) -> ("error out"=w487:errorcluster, "solar out"=w483:refnum<class "solar.lvclass">)  [unwired: 5 in]
      }
    }
    n167 = call "solar Log.vi"("error in (no error)"=w411, "DATA"=w407, "MSG"=w408, "solar in"=w410) -> ("error out"=w409:errorcluster)  [unwired: 6 in, 1 out]
  }
  n168 = call "solar Destroy.vi"("error in (no error)"=w17, "solar in"=w16) -> ()  [unwired: 9 in, 1 out]
